vi "ClearHardwareTasks.vi"(1 "Task cluster":T1={"Outbits"="Outbits", "Error Array"=[{"status"=FALSE, "code"=0, "source"=""}, {"status"=FALSE, "code"=0, "source"=""}, {"status"=FALSE, "code"=0, "source"=""}, {"status"=FALSE, "code"=0, "source"=""}, {"status"=FALSE, "code"=0, "source"=""}], "Counter"="", "Slow AO"="", "Fast AO"=[], "Trigger"=""}) -> ()   [LabVIEW 2018]
uses:
  Tasks.ctl
panel:
  # "Tasks and errors"
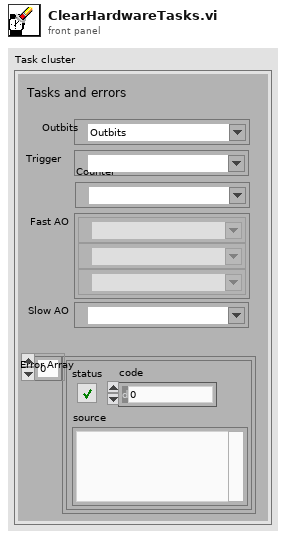
[diagram p1: front panel]
types:
  T1 = typedef "Tasks.ctl" = cluster{"Outbits":refnum<k21>, "Error Array":errorcluster[], "Counter":refnum<k21>, "Slow AO":refnum<k21>, "Fast AO":refnum<k21>[], "Trigger":refnum<k21>}
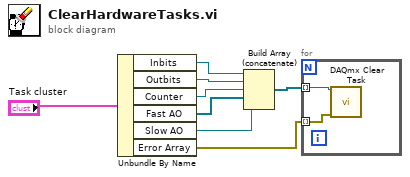
[diagram p0: block diagram]
diagram:
  n1 = Unbundle By Name("Task cluster") -> ("Inbits"=w8:refnum<k21>, "Outbits"=w7:refnum<k21>, "Counter"=w6:refnum<k21>, "Fast AO"=w5:refnum<k21>[], "Slow AO"=w4:refnum<k21>, "Error Array"=w2:errorcluster[])
  n2 = Build Array (concatenate)(w8, w7, w6, w5, w4) -> (w3:refnum<k21>[])
  n3 = for {
    tunnel: w3 -> [w10] mode=indexing
    tunnel: w2 -> [w9] mode=indexing
    n4 = call <vilib>:"DAQmx Clear Task.vi"("task in"=w10, "error in"=w9) -> ()  [unwired: 13 in, 1 out]
  }
